vi "Clear_Data_Main_v1.vi"(0 "ZI Data 0":T2, 1 "ZI Data 3":T2, 2 "Time Of Collected Data (ms)":dbl=500.0, 3 "Fixed Number Of Points":u16 min=1, 4 "Crosstalk Tolerance":dbl=0.1, 5 "error in":errorcluster, 10 "Fixed Number Of Points":bool, 12 "Check Phase Mismatch":bool) -> (9 "Trig Out Found(?)":bool, 11 "Enough Points (?)":bool, 13 "Possible Mismatch In Phase (?)":bool, 14 "Cutted Data":T1, 15 "Cutted Data 3":T1, 19 "error out":errorcluster)   [LabVIEW 2021]
uses:
  ZI_Data.ctl
  Cutted_Data.ctl
  <vilib>/Utility/error.llb/Error Cluster From Error Code.vi
  <vilib>/ErrorRing/Error Ring.xnode
  <vilib>/Analysis/NI_AALBase.lvlib
panel:
  out "first subarray":dbl[](array[numeric])
  out "subarray":dbl[](array[numeric])
  out "standard deviation 2":dbl format="%e"
  out "x*y 2":dbl
  out "x*y":dbl
  out "standard deviation":dbl format="%e"
  out "Probe Stop (s)":dbl
  out "Probe Stop (i)":i32
  out "Probe Mag Field Start (s)":dbl
  out "Probe Mag Field Start (i)":i32
  # "cutting data on demod 0 AuxIn0"
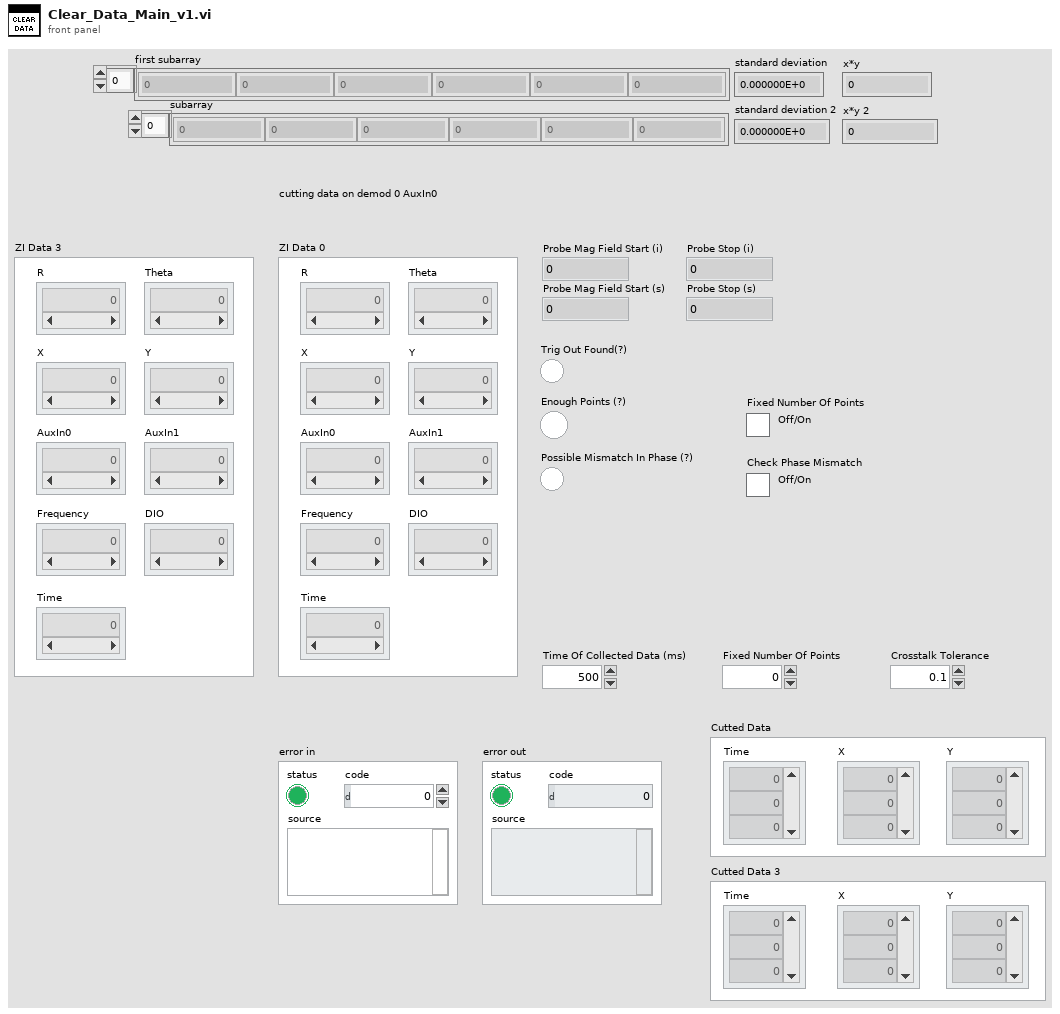
[diagram p1: front panel]
types:
  T1 = typedef "Cutted_Data.ctl" = cluster{"X":dbl[], "Y":dbl[], "Time":dbl[]}
  T2 = typedef "ZI_Data.ctl" = cluster{"R":dbl[], "Theta":dbl[], "X":dbl[], "Y":dbl[], "AuxIn0":dbl[], "AuxIn1":dbl[], "Frequency":dbl[], "DIO":dbl[], "Time":dbl[]}
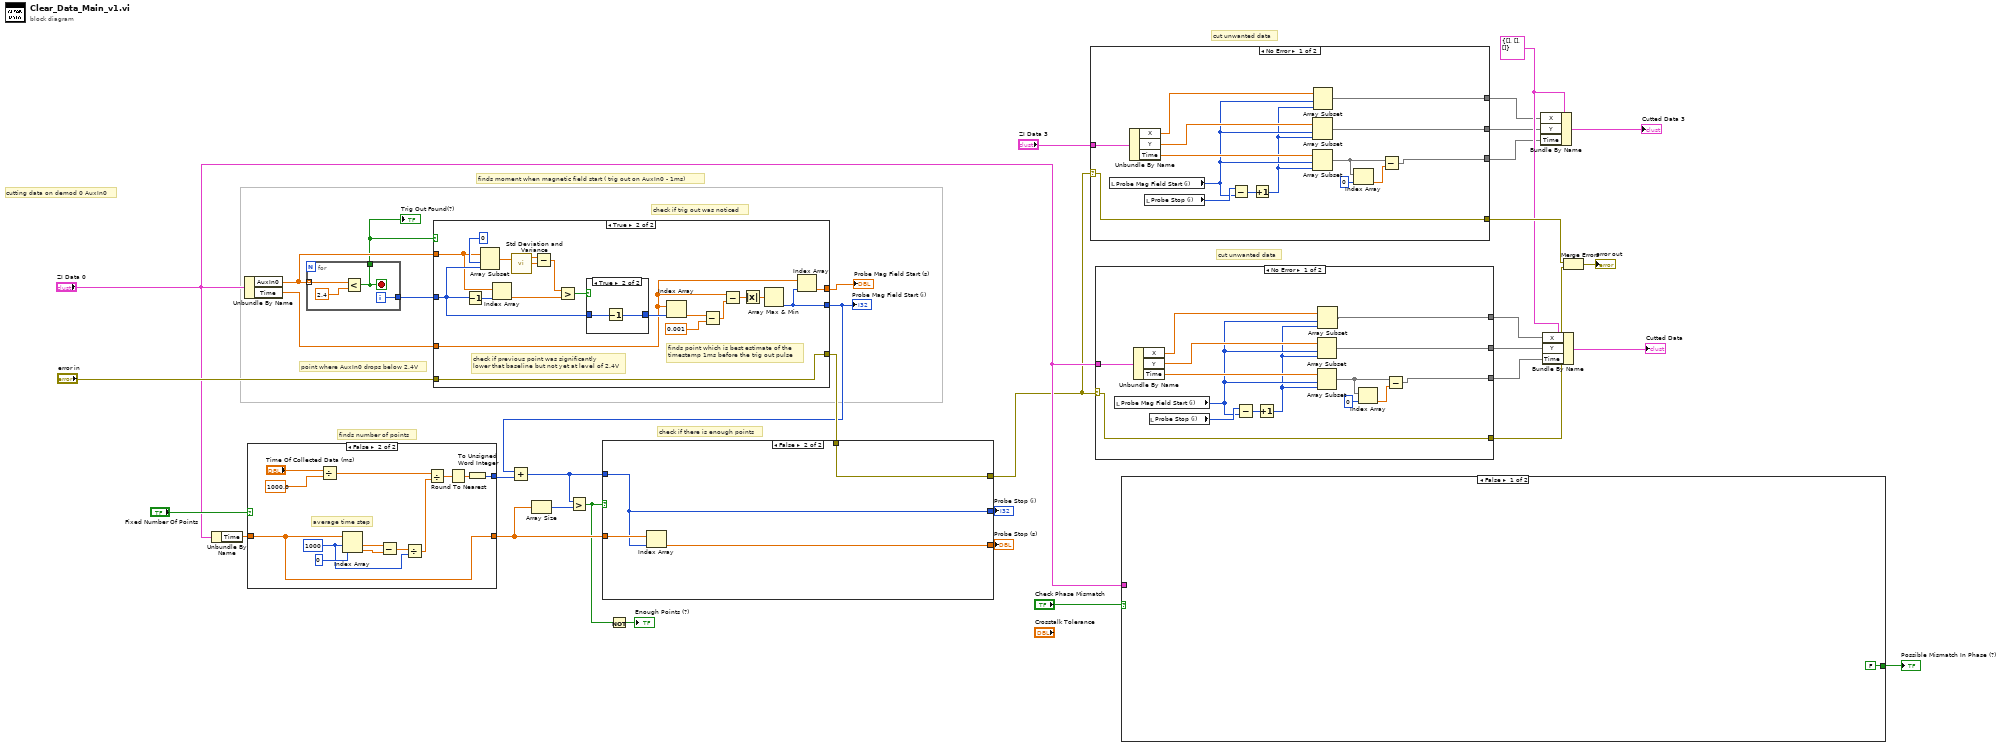
[diagram p0: block diagram]
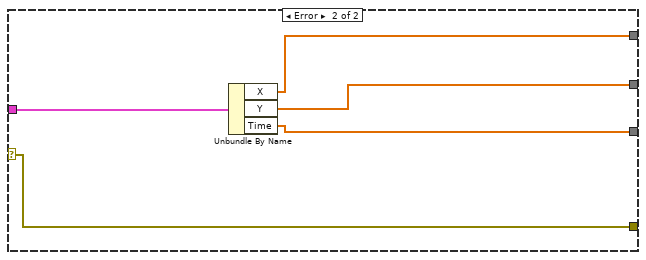
[diagram p2: hidden frame]
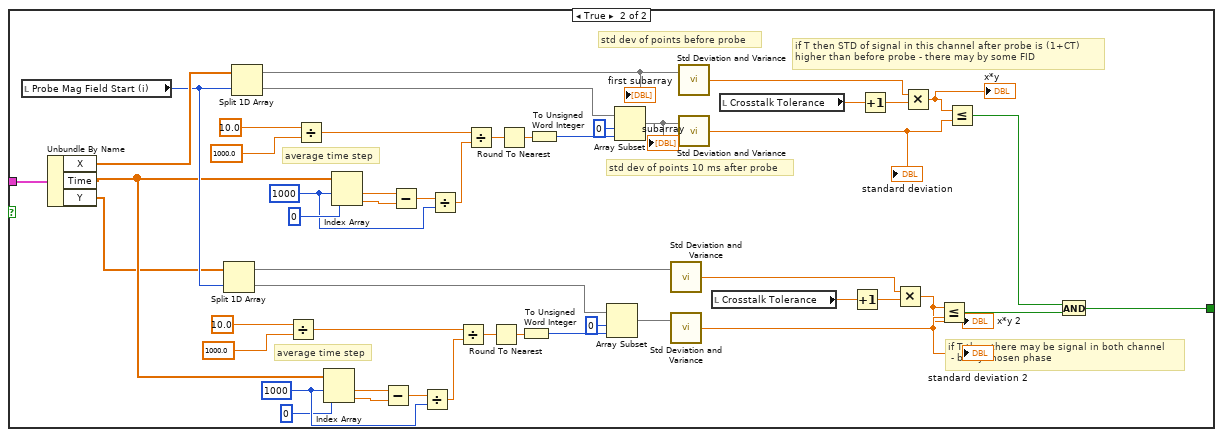
[diagram p3: hidden frame]
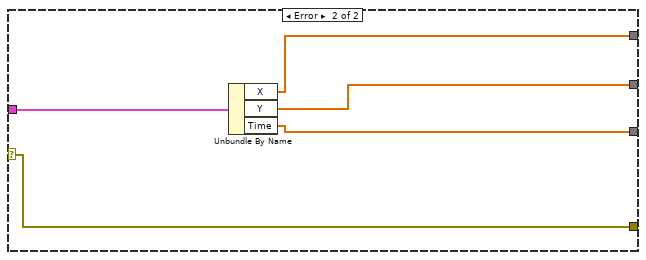
[diagram p4: hidden frame]
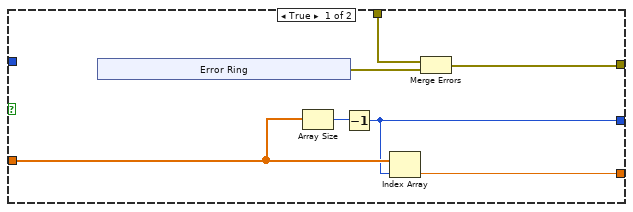
[diagram p5: hidden frame]
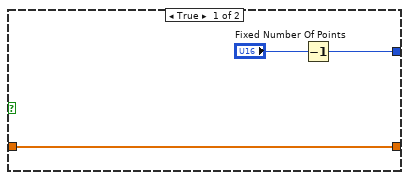
[diagram p6: hidden frame]
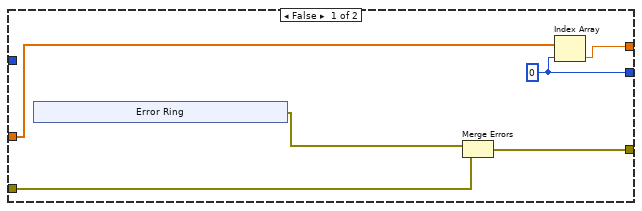
[diagram p7: hidden frame]
diagram:
  w10 = T1 {"X"=[], "Y"=[], "Time"=[]} ("Cutted Data 2")
  # "cut unwanted data"
  # "cutting data on demod 0 AuxIn0"
  # "cut unwanted data"
  # "check if there is enough points"
  # "finds number of points"
  # "check if trig out was noticed"
  # "point where AuxIn0 drops below 2.4V"
  # "finds moment when magnetic field start ( trig out on AuxIn0 - 1ms)"
  n1 = Unbundle By Name("ZI Data 0") -> ("Time"=w27:dbl[])
  n2 = Unbundle By Name("ZI Data 0") -> ("AuxIn0"=w34:dbl[], "Time"=w33:dbl[])
  n3 = case shown="False" "Fixed Number Of Points" {
    tunnel: [w36 w40] -> w28
    tunnel: w27 -> [w38 w39]
    tunnel: [w38 w39] -> w25
    frame True {
      n4 = Decrement(x="Fixed Number Of Points") -> (x-1=w36:u16)
    }
    frame False {
      w45 = 1000 ("index")
      # "average time step"
      n5 = Divide(x="Time Of Collected Data (ms)", y=1000.0) -> (x/y=w44:dbl)
      n6 = Index Array(array=w39, index #1=w45, index #2=0 ("index")) -> (element #1=w48:dbl, element #2=w47:dbl)
      n7 = Subtract(x=w48, y=w47) -> (x-y=w46:dbl)
      n8 = Divide(x=w46, y=w45) -> (x/y=w43:dbl)
      n9 = Divide(x=w44, y=w43) -> (x/y=w42:dbl)
      n10 = Round To Nearest(number=w42) -> (nearest integer value=w41:dbl)
      n11 = To Unsigned Word Integer(number=w41) -> (unsigned 16bit integer=w40:u16)
    }
  }
  n12 = for {
    tunnel: w34 -> [w55] mode=indexing
    tunnel: [w53] -> w35
    tunnel: [w52] -> w30
    i -> [w53]
    stop <- w52 stop-if-true
    n13 = Less?(x=w55, y=2.4) -> (x < y?=w52:bool)
  }
  "Trig Out Found(?)" <- w30
  n14 = case shown="True" w30 {
    tunnel: w35 -> [_ w78]
    tunnel: w34 -> [_ w76]
    tunnel: [w57 w72] -> w1
    tunnel: w33 -> [w58 w71]
    tunnel: [w56 w70] -> w32
    tunnel: "error in" -> [w61 w67]
    tunnel: [w59 w67] -> w21
    frame False {
      w57 = 0
      n15 = xnode "Error Ring"() -> ("error out"=w60:errorcluster)
      n16 = Merge Errors(w60, w61) -> (w59:errorcluster)
      n17 = Index Array(array=w58, index=w57) -> (element=w56:dbl)
    }
    frame True {
      # "finds point which is best estimate of the\ntimestamp 1ms before the trig out pulse"
      # "check if previous point was significantly\nlower that baseline but not yet at level of 2.4V"
      n18 = Decrement(x=w78) -> (x-1=w84:i32)
      n19 = Array Subset(array=w76, index=0, length=w78) -> (w85:dbl[])
      n20 = Index Array(array=w76, index=w84) -> (element=w80:dbl)
      n21 = call <vilib>:"Std Deviation and Variance.vi"("X"=w85) -> ("mean"=w83:dbl, "standard deviation"=w82:dbl)  [unwired: 1 in, 1 out]
      n22 = Subtract(x=w83, y=w82) -> (x-y=w81:dbl)
      n23 = Greater?(x=w81, y=w80) -> (0:w79:bool)
      n24 = case shown="True" w79 {
        tunnel: w78 -> [w87 w89]
        tunnel: [w87 w88] -> w77
        frame False {
        }
        frame True {
          n25 = Decrement(x=w89) -> (x-1=w88:i32)
        }
      }
      n26 = Index Array(array=w71, index=w77) -> (element=w75:dbl)
      n27 = Subtract(x=w75, y=0.001) -> (x-y=w73:dbl)
      n28 = Subtract(x=w71, y=w73) -> (x-y=w68:dbl[])
      n29 = Absolute Value(x=w68) -> (abs(x)=w69:dbl[])
      n30 = Array Max & Min(array=w69) -> (min index (indices)=w72:i32)  [unwired: 3 out]
      n31 = Index Array(array=w71, index=w72) -> (element=w70:dbl)
    }
  }
  "Probe Mag Field Start (i)" <- w1
  "Probe Mag Field Start (s)" <- w32
  n32 = Add(x=w1, y=w28) -> (x+y=w24:i32)
  n33 = Array Size(array=w25) -> (size(s)=w26:i32)
  n34 = Greater?(x=w24, y=w26) -> (0:w19:bool)
  n35 = case shown="False" w19 {
    tunnel: w25 -> [w92 w105]
    tunnel: w24 -> [_ w103]
    tunnel: [w91 w104] -> w23
    tunnel: [w90 w103] -> w22
    tunnel: w21 -> [w94 w102]
    tunnel: [w96 w102] -> w11
    frame True {
      n36 = xnode "Error Ring"() -> ("error out"=w95:errorcluster)
      n37 = Array Size(array=w92) -> (size(s)=w93:i32)
      n38 = Decrement(x=w93) -> (x-1=w90:i32)
      n39 = Index Array(array=w92, index=w90) -> (element=w91:dbl)
      n40 = Merge Errors(w94, w95) -> (w96:errorcluster)
    }
    frame False {
      n41 = Index Array(array=w105, index=w103) -> (element=w104:dbl)
    }
  }
  "Probe Stop (i)" <- w22
  "Probe Stop (s)" <- w23
  n42 = Not(x=w19) -> (.not. x?=→"Enough Points (?)":bool)
  n43 = case shown="No Error" w11 {
    selector: w11 -> [w110 w121]
    tunnel: "ZI Data 3" -> [w120 w125]
    tunnel: [w112 w124] -> w9
    tunnel: [w111 w123] -> w8
    tunnel: [w106 w122] -> w7
    tunnel: [w110 w121] -> w15
    frame No Error {
      n44 = local read "Probe Mag Field Start (i)"() -> (w114:i32)
      n45 = Unbundle By Name(w120) -> ("X"=w116:dbl[], "Y"=w115:dbl[], "Time"=w118:dbl[])
      n46 = local read "Probe Stop (i)"() -> (w119:i32)
      n47 = Subtract(x=w119, y=w114) -> (x-y=w117:i32)
      n48 = Increment(x=w117) -> (x+1=w113:i32)
      n49 = Array Subset(array=w115, index=w114, length=w113) -> (w111:dbl[])
      n50 = Array Subset(array=w118, index=w114, length=w113) -> (w109:dbl[])
      n51 = Array Subset(array=w116, index=w114, length=w113) -> (w112:dbl[])
      n52 = Index Array(array=w109, index=0) -> (element=w108:dbl)
      n53 = Subtract(x=w109, y=w108) -> (x-y=w106:dbl[])
    }
    frame Error {
      n54 = Unbundle By Name(w125) -> ("X"=w124:dbl[], "Y"=w123:dbl[], "Time"=w122:dbl[])
    }
  }
  n55 = case shown="No Error" w11 {
    selector: w11 -> [w130 w141]
    tunnel: "ZI Data 0" -> [w140 w145]
    tunnel: [w132 w144] -> w4
    tunnel: [w131 w143] -> w5
    tunnel: [w126 w142] -> w3
    tunnel: [w130 w141] -> w14
    frame No Error {
      n56 = local read "Probe Mag Field Start (i)"() -> (w134:i32)
      n57 = Unbundle By Name(w140) -> ("X"=w136:dbl[], "Y"=w135:dbl[], "Time"=w138:dbl[])
      n58 = local read "Probe Stop (i)"() -> (w139:i32)
      n59 = Subtract(x=w139, y=w134) -> (x-y=w137:i32)
      n60 = Increment(x=w137) -> (x+1=w133:i32)
      n61 = Array Subset(array=w135, index=w134, length=w133) -> (w131:dbl[])
      n62 = Array Subset(array=w138, index=w134, length=w133) -> (w129:dbl[])
      n63 = Array Subset(array=w136, index=w134, length=w133) -> (w132:dbl[])
      n64 = Index Array(array=w129, index=0) -> (element=w128:dbl)
      n65 = Subtract(x=w129, y=w128) -> (x-y=w126:dbl[])
    }
    frame Error {
      n66 = Unbundle By Name(w145) -> ("X"=w144:dbl[], "Y"=w143:dbl[], "Time"=w142:dbl[])
    }
  }
  n67 = case shown="False" "Check Phase Mismatch" {
    tunnel: "ZI Data 0" -> [_ w196]
    tunnel: [FALSE w151] -> w18
    frame False {
    }
    frame True {
      w162 = 1000 ("index")
      w190 = 1000 ("index")
      # "if T then there may be signal in both channel\n - badly chosen phase"
      # "average time step"
      # "if T then STD of signal in this channel after probe is (1+CT) \nhigher than before probe - there may by some FID"
      # "std dev of points 10 ms after probe"
      # "std dev of points before probe"
      # "average time step"
      n68 = local read "Probe Mag Field Start (i)"() -> (w156:i32)
      n69 = Unbundle By Name(w196) -> ("X"=w184:dbl[], "Time"=w155:dbl[], "Y"=w154:dbl[])
      n70 = Split 1D Array(array=w154, index=w156) -> (first subarray=w168:dbl[], second subarray=w170:dbl[])
      n71 = Split 1D Array(array=w184, index=w156) -> (first subarray=w183:dbl[], second subarray=w181:dbl[])
      "first subarray" <- w183
      n72 = Divide(x=10.0, y=1000.0) -> (x/y=w163:dbl)
      n73 = Divide(x=10.0, y=1000.0) -> (x/y=w189:dbl)
      n74 = Index Array(array=w155, index #1=w162, index #2=0 ("index")) -> (element #1=w159:dbl, element #2=w160:dbl)
      n75 = Index Array(array=w155, index #1=w190, index #2=0 ("index")) -> (element #1=w193:dbl, element #2=w192:dbl)
      n76 = Subtract(x=w159, y=w160) -> (x-y=w161:dbl)
      n77 = Subtract(x=w193, y=w192) -> (x-y=w191:dbl)
      n78 = Divide(x=w161, y=w162) -> (x/y=w164:dbl)
      n79 = Divide(x=w191, y=w190) -> (x/y=w188:dbl)
      n80 = Divide(x=w163, y=w164) -> (x/y=w165:dbl)
      n81 = Divide(x=w189, y=w188) -> (x/y=w187:dbl)
      n82 = Round To Nearest(number=w165) -> (nearest integer value=w166:dbl)
      n83 = Round To Nearest(number=w187) -> (nearest integer value=w186:dbl)
      n84 = To Unsigned Word Integer(number=w166) -> (unsigned 16bit integer=w169:u16)
      n85 = To Unsigned Word Integer(number=w186) -> (unsigned 16bit integer=w182:u16)
      n86 = Array Subset(array=w170, index=0, length=w169) -> (w171:dbl[])
      n87 = Array Subset(array=w181, index=0, length=w182) -> (w180:dbl[])
      "subarray" <- w180
      n88 = call <vilib>:"Std Deviation and Variance.vi"("X"=w168) -> ("standard deviation"=w174:dbl)  [unwired: 1 in, 2 out]
      n89 = call <vilib>:"Std Deviation and Variance.vi"("X"=w171) -> ("standard deviation"=w176:dbl)  [unwired: 1 in, 2 out]
      "standard deviation 2" <- w176
      n90 = call <vilib>:"Std Deviation and Variance.vi"("X"=w183) -> ("standard deviation"=w148:dbl)  [unwired: 1 in, 2 out]
      n91 = call <vilib>:"Std Deviation and Variance.vi"("X"=w180) -> ("standard deviation"=w177:dbl)  [unwired: 1 in, 2 out]
      "standard deviation" <- w177
      n92 = local read "Crosstalk Tolerance"() -> (w172:dbl)
      n93 = local read "Crosstalk Tolerance"() -> (w179:dbl)
      n94 = Increment(x=w172) -> (x+1=w173:dbl)
      n95 = Increment(x=w179) -> (x+1=w178:dbl)
      n96 = Multiply(x=w174, y=w173) -> (x*y=w175:dbl)
      "x*y 2" <- w175
      n97 = Multiply(x=w148, y=w178) -> (x*y=w147:dbl)
      "x*y" <- w147
      n98 = Less Or Equal?(x=w175, y=w176) -> (x <= y?=w152:bool)
      n99 = Less Or Equal?(x=w147, y=w177) -> (x <= y?=w153:bool)
      n100 = And(x=w153, y=w152) -> (x .and. y?=w151:bool)
    }
  }
  "Possible Mismatch In Phase (?)" <- w18
  n101 = Bundle By Name(cluster=w10, "X"=w9, "Y"=w8, "Time"=w7) -> (→"Cutted Data 3":T1)
  n102 = Bundle By Name(cluster=w10, "X"=w4, "Y"=w5, "Time"=w3) -> (→"Cutted Data":T1)
  n103 = Merge Errors(w15, w14) -> (→"error out":errorcluster)
